vi "Write address.vi"(8 "error in (no error)":errorcluster, 10 "address":string, 11 "IP Data Unit in":refnum<class "IP Data Unit.lvclass">) -> (0 "error out":errorcluster, 3 "IP Data Unit out":refnum<class "IP Data Unit.lvclass">)   [LabVIEW 2021, in "IP Data Unit.lvclass"]
uses:
  IP Data Unit.lvclass
  IP Data Unit.lvclass/IP Data Unit.ctl
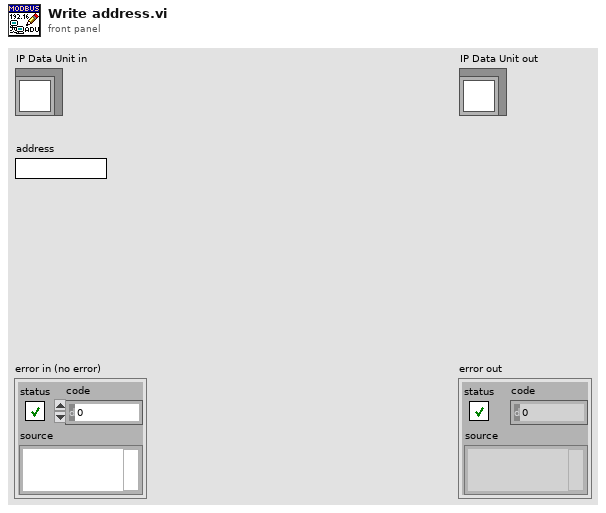
[diagram p1: front panel]
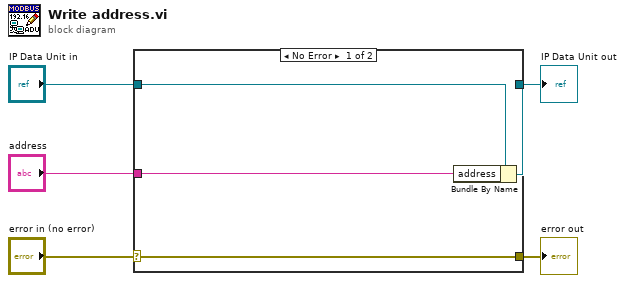
[diagram p0: block diagram]
diagram:
  n1 = case shown="No Error" "error in (no error)" {
    selector: "error in (no error)" -> [w9 w10]
    tunnel: [w9 w10] -> w4
    tunnel: [w7 w11] -> w2
    tunnel: "IP Data Unit in" -> [w8 w11]
    tunnel: "address" -> [w6 _]
    frame No Error {
      n2 = Bundle By Name(cluster=w8, "address"=w6) -> (w7:refnum<class "IP Data Unit.lvclass">)
    }
    frame Error {
    }
  }
  "error out" <- w4
  "IP Data Unit out" <- w2
